vi "最大最小值比较器（Path）.vi"(10 "reset":bool, 11 "Input":path) -> (2 "Min":path, 3 "Max":path)   [LabVIEW 2011]
doc: "功能：\n\n根据输入的数值，连续比较输入的最大值。\n\n基本算法：\n\n利用LV2全局变量（反馈节点）存储上一次输入值，和本次输入值比较，返回最大值。\n\nCSXCS_366创建"
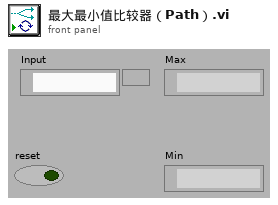
[diagram p1: front panel]
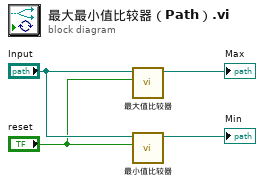
[diagram p0: block diagram]
diagram:
  n1 = call-poly "最大值比较器.vi"("reset"="reset", "Input"="Input") -> ("Max"=→"Max":path)  [unwired: 9 in]
  n2 = call-poly "最小值比较器.vi"("reset"="reset", "Input"="Input") -> ("Min"=→"Min":path)  [unwired: 9 in]
